vi "Get Selected Channels.vi"(8 "error in (no error)":errorcluster, 11 "UI in":refnum<class "UI.lvclass">) -> (0 "error out":errorcluster, 2 "Value":i32, 3 "UI out":refnum<class "UI.lvclass">)   [LabVIEW 2015, in "UI.lvlib" / "UI.lvclass"]
uses:
  UI.lvclass
  UI.lvclass/UI.ctl
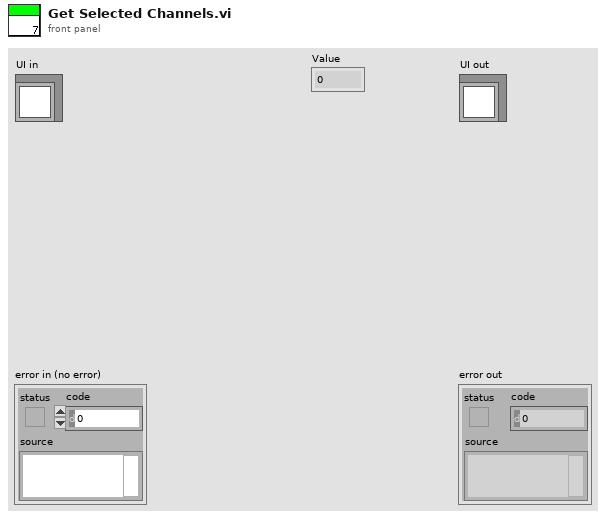
[diagram p1: front panel]
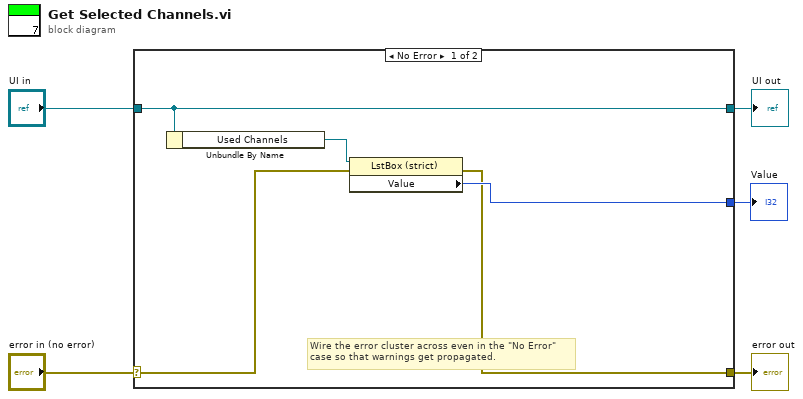
[diagram p0: block diagram]
diagram:
  n1 = case shown="No Error" "error in (no error)" {
    selector: "error in (no error)" -> [w7 w12]
    tunnel: [w6 w12] -> w4
    tunnel: [w10 w11] -> w2
    tunnel: "UI in" -> [w10 w11]
    tunnel: [w8 _] -> w1
    frame No Error {
      # "Wire the error cluster across even in the \"No Error\"\ncase so that warnings get propagated."
      n2 = Unbundle By Name(w10) -> ("Used Channels"=w9:refnum<vi>)
      n3 = property class="LstBox (strict)"(reference=w9, error in=w7) -> (error out=w6:errorcluster, "Value"=w8:i32)  [unwired: 1 out]
    }
    frame Error {
    }
  }
  "error out" <- w4
  "UI out" <- w2
  "Value" <- w1
